vi "Scott's mean filter!.vi"(8 "window size":i32, 11 "input":dbl[](array[numeric])) -> (3 "output":dbl[](array[numeric]))   [LabVIEW 2025]
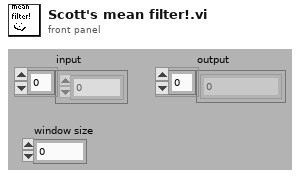
[diagram p1: front panel]
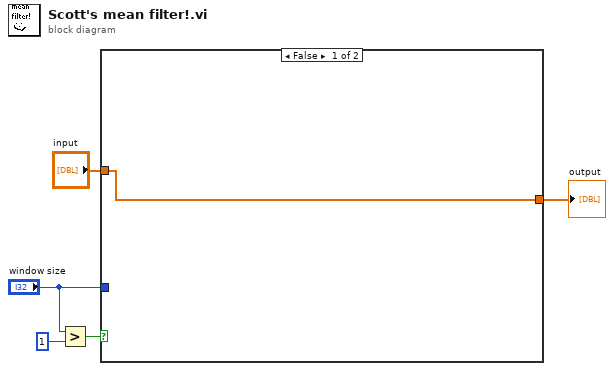
[diagram p0: block diagram]
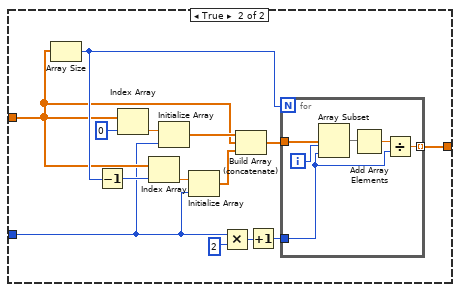
[diagram p2: hidden frame]
diagram:
  n1 = Greater?(x="window size", y=1) -> (0:w3:bool)
  n2 = case shown="False" w3 {
    tunnel: [w6 w20] -> w5
    tunnel: "input" -> [w6 w13]
    tunnel: "window size" -> [_ w8]
    frame False {
    }
    frame True {
      n3 = Array Size(array=w13) -> (size(s)=w16:i32)
      n4 = Decrement(x=w16) -> (x-1=w15:i32)
      n5 = Index Array(array=w13, index=0) -> (element=w18:dbl)
      n6 = Index Array(array=w13, index=w15) -> (element=w17:dbl)
      n7 = Initialize Array(w18, w8) -> (w14:dbl[])
      n8 = Initialize Array(w17, w8) -> (w12:dbl[])
      n9 = Multiply(x=w8, y=2) -> (x*y=w10:i32)
      n10 = Build Array (concatenate)(w14, w13, w12) -> (w11:dbl[])
      n11 = Increment(x=w10) -> (x+1=w7:i32)
      n12 = for {
        N: w16 -> [_]
        tunnel: w11 -> [w26]
        tunnel: [w21] -> w20 mode=indexing
        tunnel: w7 -> [w22]
        i -> [w23]
        n13 = Array Subset(array=w26, index=w23, length=w22) -> (w25:dbl[])
        n14 = Add Array Elements(numeric array=w25) -> (sum=w24:dbl)
        n15 = Divide(x=w24, y=w22) -> (x/y=w21:dbl)
      }
    }
  }
  "output" <- w5
